vi "subAcquisition_StreamMovie.vi"(4 "Elapsed time (sec) Refnum":refnum<vi>, 6 "Frames Recorded Refnum":refnum<vi>, 7 "File path":path, 8 "error in (no error)":errorcluster, 9 "Movie frame rate (Hz)":dbl=1000.0 format="%0.0f", 10 "# frames":u32=1000, 11 "Handle in":u32) -> (0 "error out":errorcluster, 3 "Handle out":u32)   [LabVIEW 2015]
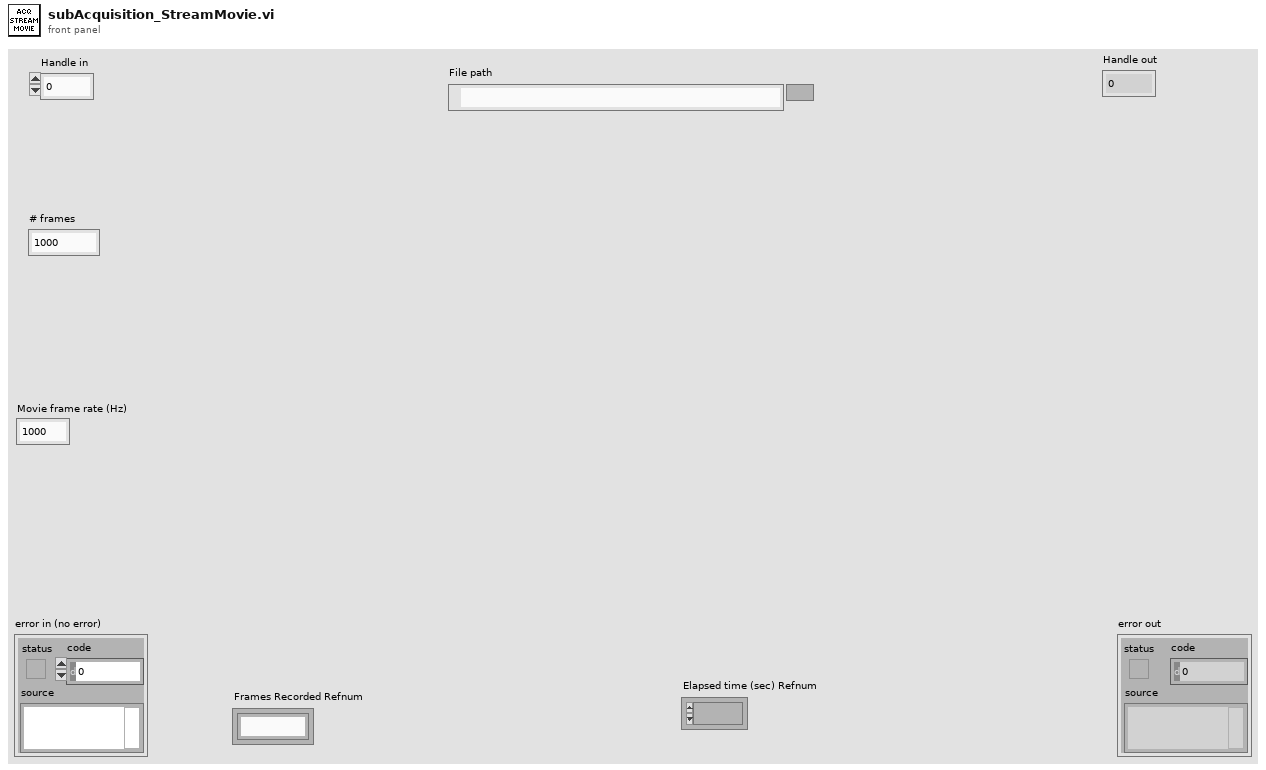
[diagram p1: front panel]
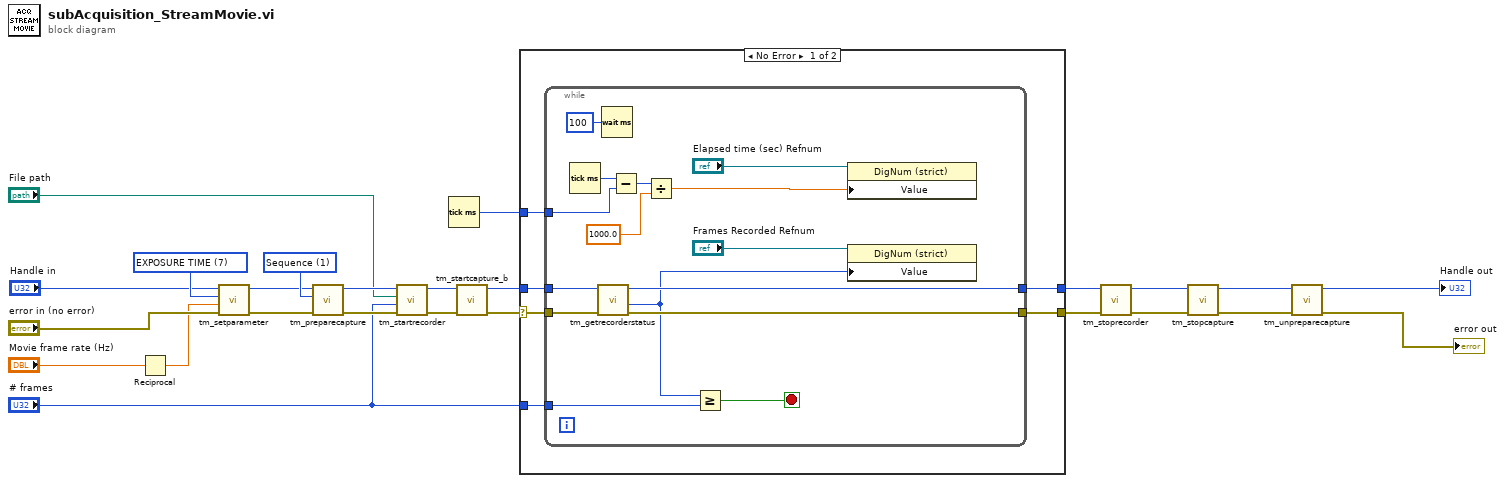
[diagram p0: block diagram]
diagram:
  w8 = 7 items=["BINNING"=1, "BITS PER CHANNEL"=2, "ACTIVE VIEW INDEX"=3, "CCD MODE"=4, "SENSOR MODE"=5, "READOUT MODE"=6, "EXPOSURE TIME"=7, "CONTRAST GAIN"=8, "CONTRAST OFFSET"=9, "LIGHT MODE"=10, "SENSITIVITY"=11, "WHITE BALANCE"=12, "PHOTON IMAGING MODE"=13, "HIGH DYNAMIC RANGE MODE"=14, "TRIGGER SOURCE"=15, "TRIGGER ACTIVE"=16, "TRIGGER MODE"=17, "TRIGGER POLARITY"=18, "TRIGGER GLOBAL EXPOSURE"=19, "FIRST TRIGGER BEHAVIOR"=20, "TRIGGER TIMES"=21, "OUTPUT TRIGGER POLARITY"=22, "OUTPUT TRIGGER DELAY"=23, "OUTPUT TRIGGER PERIOD"=24, "TEMPERATURE"=25, "TEMPERATURE TARGET"=26, "SENSOR COOLER FAN"=27, "MECHANICAL SHUTTER"=28, "BACK FOCUS POSITION"=29, "FRAMEBUNDLE MODE"=30, "FRAMEBUNDLE NUMBER"=31, "LINEBUNDLE HEIGHT"=32, "TRIGGER CONNECTOR"=33, "IMAGE PIXEL TYPE"=34] ("Parameter")
  w25 = 1 items=["Snap", "Sequence"] ("Capture mode")
  n1 = Reciprocal(x="Movie frame rate (Hz)") -> (1/x=w3:dbl)
  n2 = call "tm_setparameter.vi"("error in (no error)"="error in (no error)", "Value in"=w3, "Parameter"=w8, "Handle in"="Handle in") -> ("error out"=w6:errorcluster, "Handle out"=w7:u32)  [unwired: 6 in]
  n3 = call "tm_preparecapture.vi"("error in (no error)"=w6, "Capture mode"=w25, "Handle in"=w7) -> ("error out"=w24:errorcluster, "Handle out"=w23:u32)  [unwired: 5 in, 2 out]
  n4 = call "tm_startrecorder.vi"("error in (no error)"=w24, "frames"="# frames", "File"="File path", "Handle in"=w23) -> ("error out"=w22:errorcluster, "Handle out"=w21:u32)  [unwired: 6 in]
  n5 = Tick Count (ms)() -> (millisecond timer value=w12:u32)
  n6 = call "tm_startcapture_b.vi"("error in (no error)"=w22, "Handle in"=w21) -> ("error out"=w20:errorcluster, "Handle out"=w19:u32)  [unwired: 8 in]
  n7 = case shown="No Error" w20 {
    selector: w20 -> [w31 w47]
    tunnel: w19 -> [w30 w48]
    tunnel: [w28 w48] -> w13
    tunnel: [w29 w47] -> w14
    tunnel: "# frames" -> [w27 _]
    tunnel: w12 -> [w26 _]
    frame No Error {
      n8 = while {
        tunnel: w31 -> [w44]
        tunnel: w30 -> [w43]
        tunnel: [w42] -> w29
        tunnel: [w45] -> w28
        tunnel: w27 -> [w46]
        tunnel: w26 -> [w38]
        stop <- w41 stop-if-true
        n9 = Tick Count (ms)() -> (millisecond timer value=w37:u32)
        n10 = call "tm_getrecorderstatus.vi"("error in (no error)"=w44, "Handle"=w43) -> ("error out"=w42:errorcluster, "Count"=w32:i32, "Handle"=w45:u32)  [unwired: 6 in, 1 out]
        n11 = Wait (ms)(milliseconds to wait=u32 100) -> ()  [unwired: 1 out]
        n12 = Subtract(x=w37, y=w38) -> (x-y=w36:u32)
        n13 = Divide(x=w36, y=1000.0) -> (x/y=w34:dbl)
        n14 = Greater Or Equal?(x=w32, y=w46) -> (x >= y?=w41:bool)
        n15 = property class="DigNum (strict)"(reference="Elapsed time (sec) Refnum", "Value"=w34) -> ()  [unwired: 1 in, 2 out]
        n16 = property class="DigNum (strict)"(reference="Frames Recorded Refnum", "Value"=w32) -> ()  [unwired: 1 in, 2 out]
      }
    }
    frame Error {
    }
  }
  n17 = call "tm_stoprecorder.vi"("error in (no error)"=w14, "Handle in"=w13) -> ("error out"=w15:errorcluster, "Handle out"=w16:u32)  [unwired: 8 in]
  n18 = call "tm_stopcapture.vi"("error in (no error)"=w15, "Handle in"=w16) -> ("error out"=w18:errorcluster, "Handle out"=w17:u32)  [unwired: 8 in]
  n19 = call "tm_unpreparecapture.vi"("error in (no error)"=w18, "Handle in"=w17) -> ("error out"=→"error out":errorcluster, "Handle out"=→"Handle out":u32)  [unwired: 8 in]
